vi "serialize.vi"() -> ()   [LabVIEW 2013, in "tag bus tests.lvlib"]
uses:
  tag bus tests.lvlib
  tag/Data Type.ctl
  tag/data bus tag description.lvclass
  tag/data bus tag description.lvclass/data bus tag description.ctl
  tag/read data type.vi
  tag/read metadata.vi
  tag/read tag name.vi
  tag/read raw default value.vi
panel:
  out "Array 2":bool[](array[boolean])
  out "x = y? 4":bool
  out "x = y? 3":bool
  out "x = y? 2":bool
  out "x = y?":bool
  out "data type 2":T1
  out "metadata 2":string
  out "name 2":string
  out "unformatted default 2":variant
  out "unformatted default":variant
  out "name":string
  out "metadata":string
  out "data type":T1
  out "ok":bool
  out "Array":bool[](array[boolean])
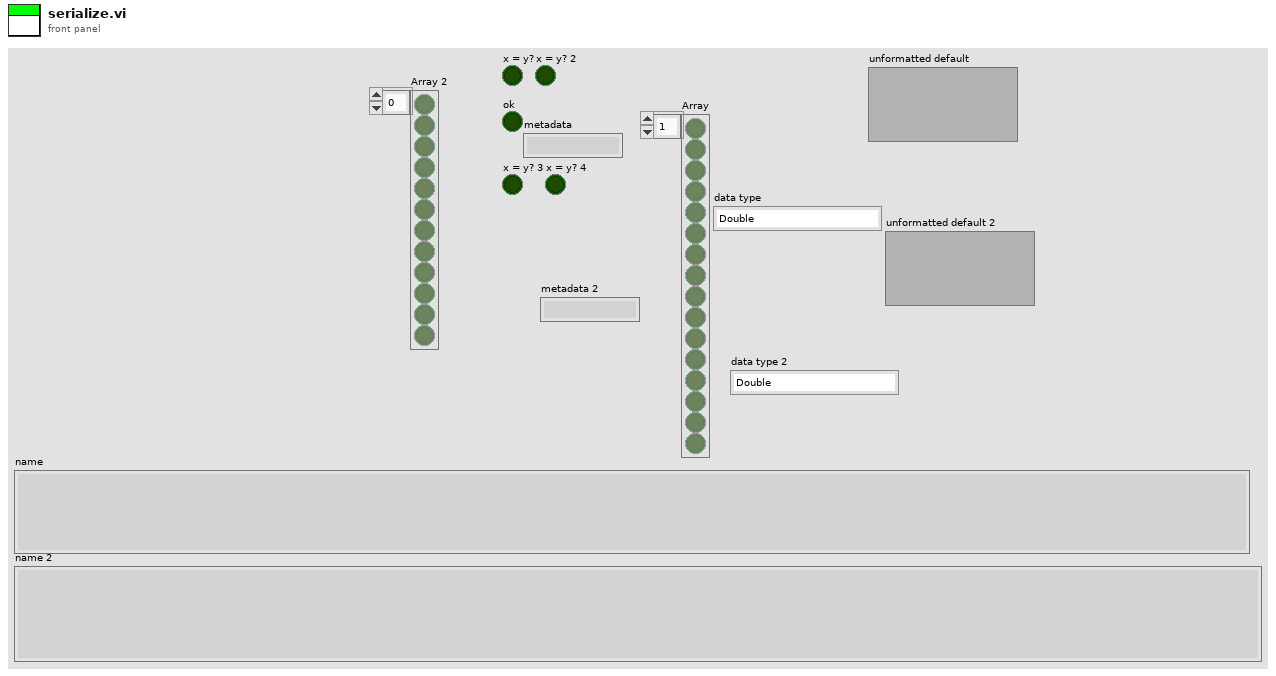
[diagram p1: front panel]
types:
  T1 = typedef "data bus tag description.lvclass/Data Type.ctl" = enum16{"Double", "I64", "Boolean", "Array of Double", "Array of I64", "Variant"}
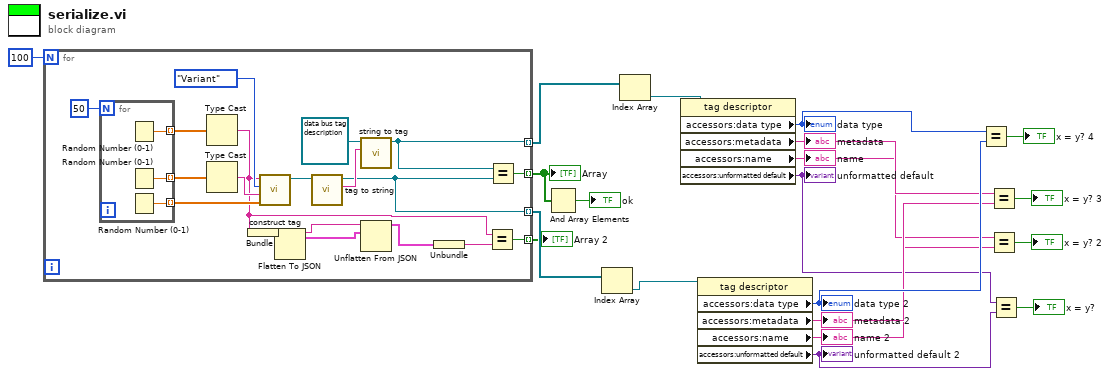
[diagram p0: block diagram]
diagram:
  n1 = for {
    N: 100 -> [_]
    tunnel: [w31] -> w19 mode=indexing
    tunnel: [w28] -> w16 mode=indexing
    tunnel: [w27] -> w17 mode=indexing
    tunnel: [w21] -> w1 mode=indexing
    n2 = for {
      N: 50 -> [_]
      tunnel: [w41] -> w36 mode=indexing
      tunnel: [w40] -> w37 mode=indexing
      tunnel: [w39] -> w30 mode=indexing
      n3 = Random Number (0-1)() -> (number: 0 to 1=w40:dbl)
      n4 = Random Number (0-1)() -> (number: 0 to 1=w41:dbl)
      n5 = Random Number (0-1)() -> (number: 0 to 1=w39:dbl)
    }
    n6 = Type Cast(x=w37) -> (*(type *) &x=w22:string)  [unwired: 1 in]
    n7 = Type Cast(x=w36) -> (*(type *) &x=w35:string)  [unwired: 1 in]
    n8 = Bundle(w22) -> (w25:cluster{string})  [unwired: 1 in]
    n9 = call "construct tag.vi"("raw default"=w30, "metadata"=w35, "data type"=Data_Type."Variant", "name"=w22) -> ("system tag out"=w34:refnum<class "data bus tag description.lvclass">)  [unwired: 7 in]
    n10 = Flatten To JSON(anything=w25) -> (JSON string=w26:string)  [unwired: 2 in, 1 out]
    n11 = call "tag to string.vi"("tag descriptor in"=w34) -> ("tag string"=w33:string, "tag descriptor out"=w27:refnum<class "data bus tag description.lvclass">)  [unwired: 8 in, 1 out]
    n12 = call "string to tag.vi"("tag string"=w33, "tag descriptor in"=refnum<class "data bus tag description.lvclass"> refnum) -> ("tag descriptor out"=w28:refnum<class "data bus tag description.lvclass">)  [unwired: 8 in, 1 out]
    n13 = Unflatten From JSON(JSON string=w26, type and defaults=w25) -> (value=w24:cluster{string})  [unwired: 5 in, 1 out]
    n14 = Unbundle(w24) -> (w23:string)
    n15 = Equal?(x=w22, y=w23) -> (x = y?=w21:bool)
    n16 = Equal?(x=w28, y=w27) -> (x = y?=w31:bool)
  }
  "Array" <- w19
  "Array 2" <- w1
  n17 = And Array Elements(Boolean array=w19) -> (logical AND=→"ok":bool)
  n18 = Index Array(array=w17) -> (element=w14:refnum<class "data bus tag description.lvclass">)  [unwired: 1 in]
  n19 = Index Array(array=w16) -> (element=w15:refnum<class "data bus tag description.lvclass">)  [unwired: 1 in]
  n20 = property class="tag descriptor"(reference=w15) -> ("accessors:data type"=w13:T1, "accessors:metadata"=w11:string, "accessors:name"=w9:string, "accessors:unformatted default"=w7:variant)  [unwired: 1 in, 2 out]
  "data type" <- w13
  "metadata" <- w11
  "name" <- w9
  "unformatted default" <- w7
  n21 = property class="tag descriptor"(reference=w14) -> ("accessors:data type"=w12:T1, "accessors:metadata"=w10:string, "accessors:name"=w8:string, "accessors:unformatted default"=w6:variant)  [unwired: 1 in, 2 out]
  "data type 2" <- w12
  "metadata 2" <- w10
  "name 2" <- w8
  "unformatted default 2" <- w6
  n22 = Equal?(x=w13, y=w12) -> (x = y?=→"x = y? 4":bool)
  n23 = Equal?(x=w11, y=w10) -> (x = y?=→"x = y? 3":bool)
  n24 = Equal?(x=w9, y=w8) -> (x = y?=→"x = y? 2":bool)
  n25 = Equal?(x=w7, y=w6) -> (x = y?=→"x = y?":bool)
